vi "Layout Controls.vi"(7 "Control Cliuster":refnum<vi>, 8 "error out":errorcluster, 9 "NewBnds":T2, 10 "Waveform Ref":refnum<vi>, 11 "Controls Refs":T1) -> (0 "error out 2":errorcluster)   [LabVIEW 2011, in "Waveform Control.xctl"]
uses:
  Waveform Control.xctl
  <vilib>/Utility/miscctls.llb/LVRectTypeDef.ctl
  <vilib>/Utility/miscctls.llb/LVPositionTypeDef.ctl
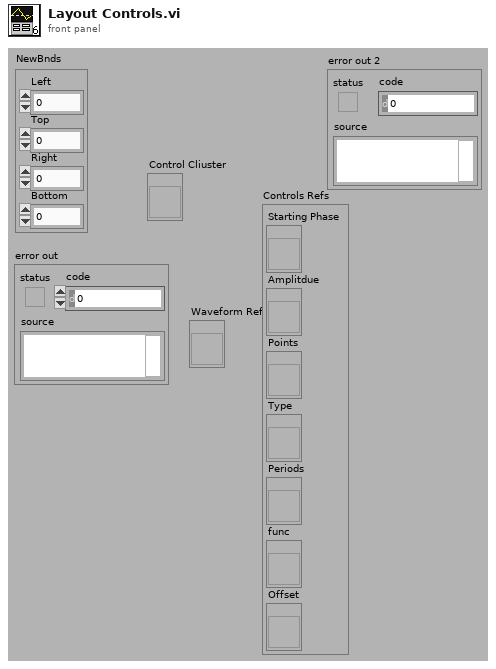
[diagram p1: front panel]
types:
  T1 = cluster{"Starting Phase":refnum<vi>, "Amplitdue":refnum<vi>, "Points":refnum<vi>, "Type":refnum<vi>, "Periods":refnum<vi>, "func":refnum<vi>, "Offset":refnum<vi>}
  T2 = typedef "LVRectTypeDef.ctl" = cluster{"Left":i16, "Top":i16, "Right":i16, "Bottom":i16}
  T3 = typedef "LVPositionTypeDef.ctl" = cluster{"Left":i32, "Top":i32}
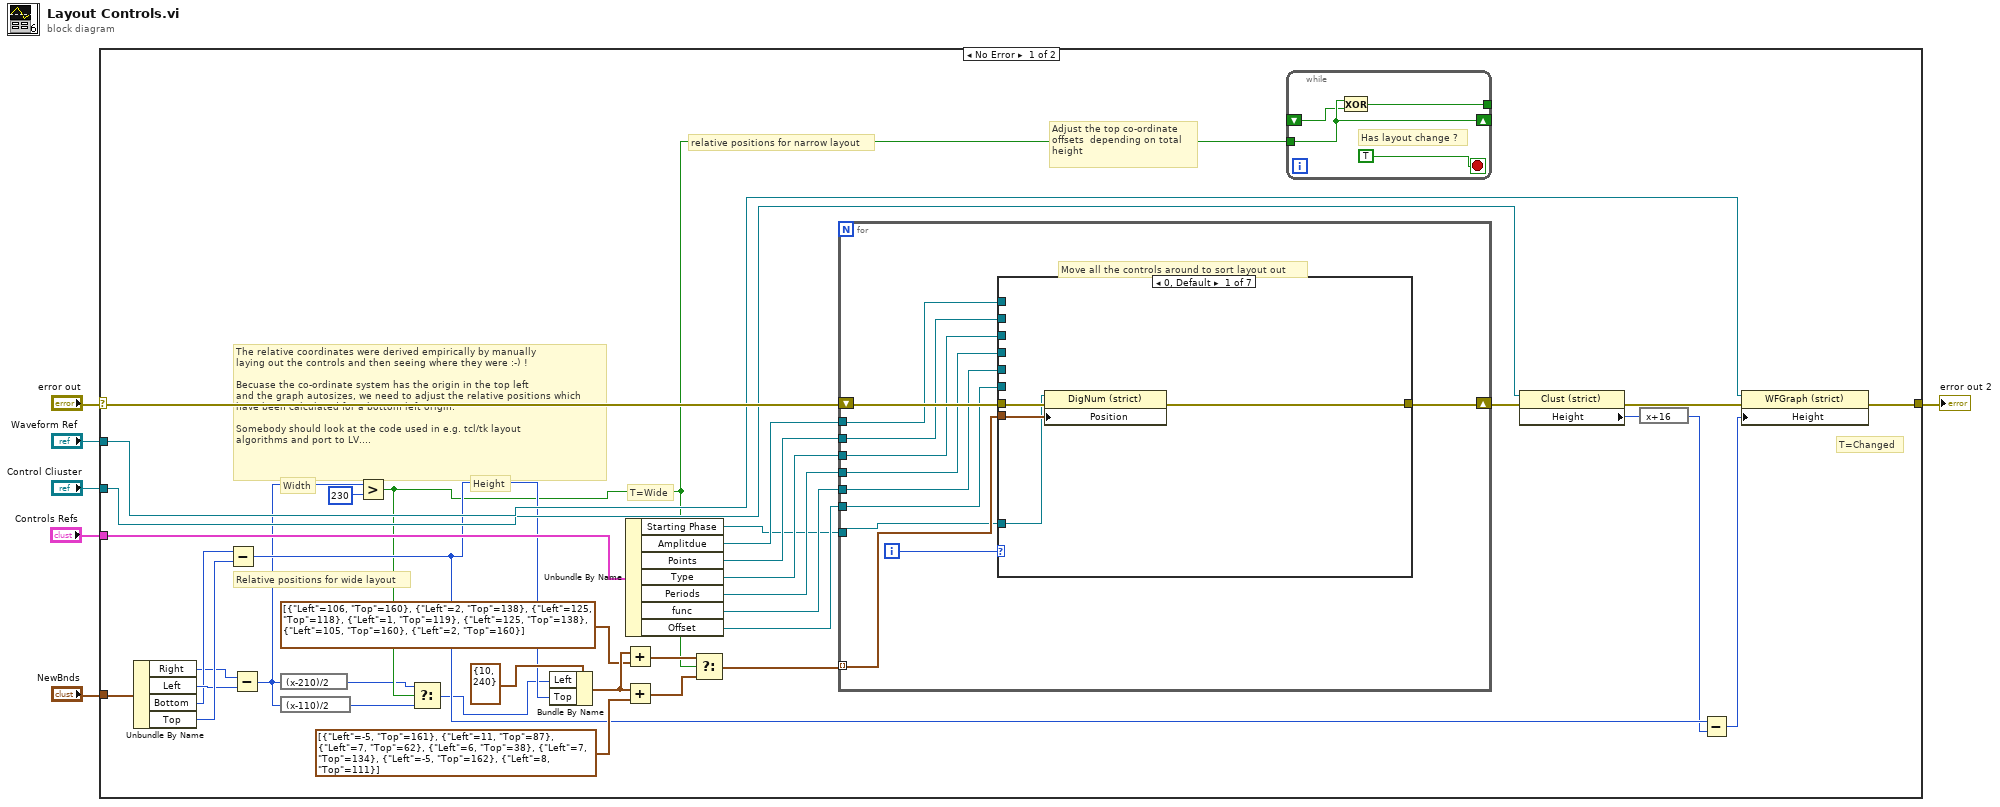
[diagram p0: block diagram]
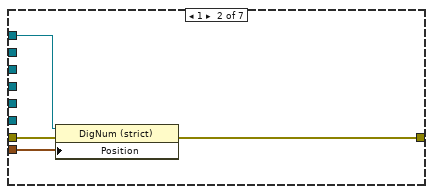
[diagram p2: hidden frame]
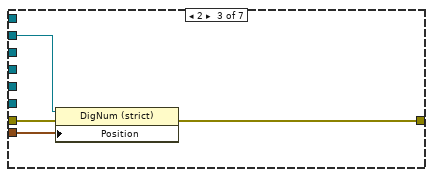
[diagram p3: hidden frame]
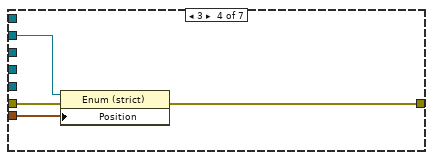
[diagram p4: hidden frame]
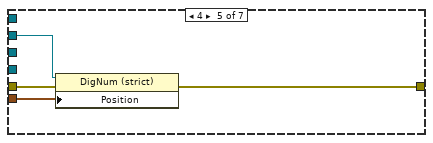
[diagram p5: hidden frame]
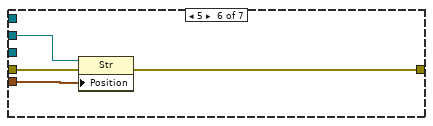
[diagram p6: hidden frame]
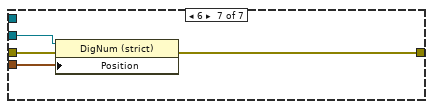
[diagram p7: hidden frame]
diagram:
  n1 = case shown="No Error" "error out" {
    selector: "error out" -> [w42 w86]
    tunnel: [w41 w86] -> w5
    tunnel: "NewBnds" -> [w27 _]
    tunnel: "Waveform Ref" -> [w26 _]
    tunnel: "Controls Refs" -> [w25 _]
    tunnel: "Control Cliuster" -> [w17 _]
    frame No Error {
      # "The relative coordinates were derived empirically by manually \nlaying out the controls and then seeing where they were :-) !\n\nBecuase the co-ordinate system has the origin in the top left\nand the graph autosizes, we need to adjust the relative positions which\nhave been calculated for a bottom left origin.\n\nSomebody should look at the code used in e.g. tcl/tk layout\nalgorithms and port to LV...."
      # "Adjust the top co-ordinate \noffsets  depending on total \nheight"
      # "T=Changed"
      # "relative positions for narrow layout"
      # "Relative positions for wide layout"
      # "T=Wide"
      # "Height"
      # "Width"
      n2 = Unbundle By Name(w27) -> ("Right"=w35:i16, "Left"=w37:i16, "Bottom"=w36:i16, "Top"=w38:i16)
      n3 = Subtract(x=w36, y=w38) -> (x-y=w15:i16)
      n4 = Subtract(x=w35, y=w37) -> (x-y=w8:i16)
      n5 = expression code="(x-210)/2"(w8) -> (w10:i16)
      n6 = expression code="(x-110)/2"(w8) -> (w9:i16)
      n7 = Greater?(x=w8, y=i16 230) -> (0:w11:bool)
      n8 = Select(t=w10, s=w11, f=w9) -> (s? t:f=w7:i16)
      n9 = Bundle By Name(cluster=T3 {"Left"=10, "Top"=240} ("Position"), "Left"=w7, "Top"=w15) -> (w39:T3)
      n10 = Add(x=w39, y=T3[] [{"Left"=106, "Top"=160}, {"Left"=2, "Top"=138}, {"Left"=125, "Top"=118}, {"Left"=1, "Top"=119}, {"Left"=125, "Top"=138}, {"Left"=105, "Top"=160}, {"Left"=2, "Top"=160}] ("appended array")) -> (x+y=w32:T3[])
      n11 = Add(x=w39, y=T3[] [{"Left"=-5, "Top"=161}, {"Left"=11, "Top"=87}, {"Left"=7, "Top"=62}, {"Left"=6, "Top"=38}, {"Left"=7, "Top"=134}, {"Left"=-5, "Top"=162}, {"Left"=8, "Top"=111}] ("appended array")) -> (x+y=w31:T3[])
      n12 = Unbundle By Name(w25) -> ("Starting Phase"=w18:refnum<vi>, "Amplitdue"=w24:refnum<vi>, "Points"=w23:refnum<vi>, "Type"=w22:refnum<vi>, "Periods"=w21:refnum<vi>, "func"=w20:refnum<vi>, "Offset"=w19:refnum<vi>)
      n13 = Select(t=w32, s=w11, f=w31) -> (s? t:f=w30:T3[])
      n14 = for {
        tunnel: w30 -> [w52] mode=indexing
        shift-right: [w51] -> w40
        shift-left: w42 -> [w50]
        tunnel: w18 -> [w49]
        tunnel: w24 -> [w48]
        tunnel: w23 -> [w47]
        tunnel: w22 -> [w46]
        tunnel: w21 -> [w45]
        tunnel: w20 -> [w44]
        tunnel: w19 -> [w43]
        i -> [w53]
        # "Move all the controls around to sort layout out"
        n15 = case shown="0, Default" w53 {
          tunnel: w52 -> [w57 w61 w65 w69 w73 w77 w81]
          tunnel: [w56 w59 w63 w67 w71 w75 w79] -> w51
          tunnel: w50 -> [w55 w60 w64 w68 w72 w76 w80]
          tunnel: w49 -> [w54 _ _ _ _ _ _]
          tunnel: w48 -> [_ w58 _ _ _ _ _]
          tunnel: w47 -> [_ _ w62 _ _ _ _]
          tunnel: w46 -> [_ _ _ w66 _ _ _]
          tunnel: w45 -> [_ _ _ _ w70 _ _]
          tunnel: w44 -> [_ _ _ _ _ w74 _]
          tunnel: w43 -> [_ _ _ _ _ _ w78]
          frame 0, Default {
            n16 = property on="Property Node" class="DigNum (strict)"(reference=w54, error in=w55, "Position"=w57) -> (error out=w56:errorcluster)  [unwired: 1 out]
          }
          frame 1 {
            n17 = property on="Property Node" class="DigNum (strict)"(reference=w58, error in=w60, "Position"=w61) -> (error out=w59:errorcluster)  [unwired: 1 out]
          }
          frame 2 {
            n18 = property on="Property Node" class="DigNum (strict)"(reference=w62, error in=w64, "Position"=w65) -> (error out=w63:errorcluster)  [unwired: 1 out]
          }
          frame 3 {
            n19 = property on="Property Node" class="Enum (strict)"(reference=w66, error in=w68, "Position"=w69) -> (error out=w67:errorcluster)  [unwired: 1 out]
          }
          frame 4 {
            n20 = property on="Property Node" class="DigNum (strict)"(reference=w70, error in=w72, "Position"=w73) -> (error out=w71:errorcluster)  [unwired: 1 out]
          }
          frame 5 {
            n21 = property on="Property Node" class="Str"(reference=w74, error in=w76, "Position"=w77) -> (error out=w75:errorcluster)  [unwired: 1 out]
          }
          frame 6 {
            n22 = property on="Property Node" class="DigNum (strict)"(reference=w78, error in=w80, "Position"=w81) -> (error out=w79:errorcluster)  [unwired: 1 out]
          }
        }
      }
      n23 = while {
        shift-right: [w84] -> _
        shift-left: _ -> [w83]
        tunnel: w11 -> [w84]
        tunnel: [w82] -> _
        stop <- TRUE stop-if-true
        # "Has layout change ?"
        n24 = Exclusive Or(1:w83, 2:w84) -> (0:w82:bool)
      }
      n25 = property on="Property Node" class="Clust (strict)"(reference=w17, error in=w40) -> (error out=w16:errorcluster, "Height"=w14:u32)  [unwired: 1 out]
      n26 = expression code="x+16"(w14) -> (w12:u32)
      n27 = Subtract(x=w15, y=w12) -> (x-y=w13:u32)
      n28 = property on="Property Node" class="WFGraph (strict)"(reference=w26, error in=w16, "Height"=w13) -> (error out=w41:errorcluster)  [unwired: 1 out]
    }
    frame Error {
    }
  }
  "error out 2" <- w5
